vi "OpenCPClior.vi"(11 "CPC port":refnum<visa-resource-name>="COM1") -> (2 "CPC model":string, 3 "dup CPC port":refnum<visa-resource-name>, 10 "read buffer":string)   [LabVIEW 2017]
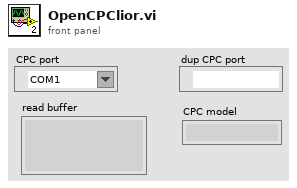
[diagram p1: front panel]
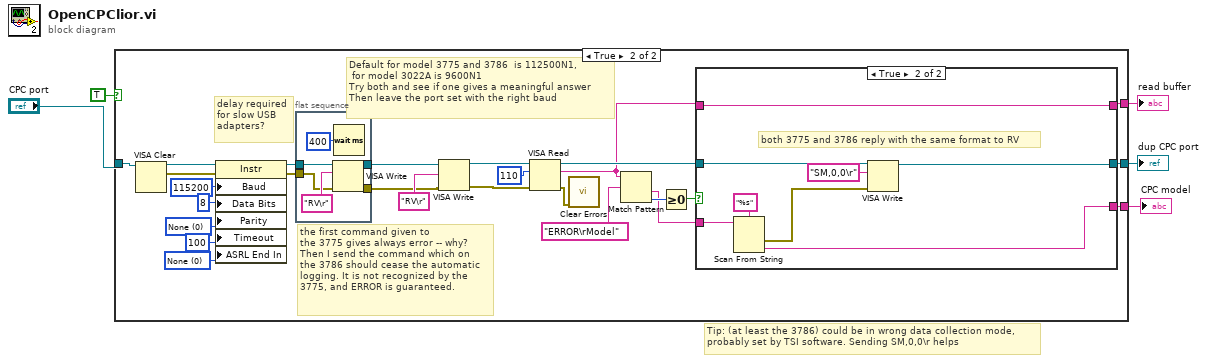
[diagram p0: block diagram]
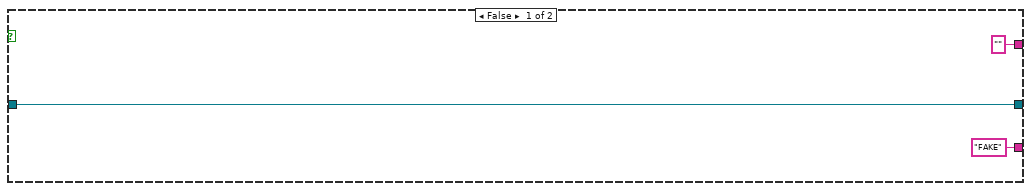
[diagram p2: hidden frame]
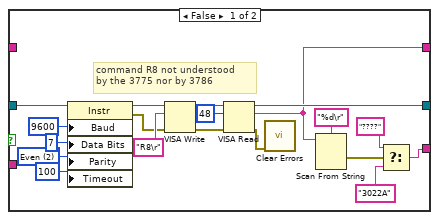
[diagram p3: hidden frame]
diagram:
  # "Tip: (at least the 3786) could be in wrong data collection mode,\nprobably set by TSI software. Sending SM,0,0\\r helps"
  n1 = case shown="True" TRUE {
    tunnel: ["FAKE" ("y") w32] -> w5
    tunnel: ["" ("read buffer") w29] -> w4
    tunnel: "CPC port" -> [w8 w26]
    tunnel: [w8 w25] -> w3
    frame False {
    }
    frame True {
      w9 = u16 0 items=["None", "Last Bit", "TermChar"] ("Serial Settings:End Mode for Reads")
      w19 = u16 0 items=["None", "Odd", "Even", "Mark", "Space"] ("Serial Settings:Parity")
      # "delay required\nfor slow USB\nadapters?"
      # "the first command given to\nthe 3775 gives always error -- why?\nThen I send the command which on\nthe 3786 should cease the automatic\nlogging. It is not recognized by the\n3775, and ERROR is guaranteed."
      # "Default for model 3775 and 3786  is 112500N1,\n for model 3022A is 9600N1\nTry both and see if one gives a meaningful answer\nThen leave the port set with the right baud"
      n2 = VISA Clear(VISA resource name=w26) -> (VISA resource name out=w22:refnum<visa-resource-name>, error out=w17:errorcluster)  [unwired: 1 in]
      n3 = property class="Instr"(reference=w22, error in=w17, "Baud"=u32 115200 ("Serial Settings:Baud Rate"), "Data Bits"=u16 8 ("Serial Settings:Data Bits"), "Parity"=w19, "Timeout"=u32 100 ("General Settings:Timeout Value"), "ASRL End In"=w9) -> (reference out=w23:refnum<visa-resource-name>, error out=w16:errorcluster)
      n4 = flat-sequence {
        tunnel: [w40] -> w24
        tunnel: w23 -> [w38]
        tunnel: w16 -> [w37]
        tunnel: [w36] -> w15
        frame #0 {
          n5 = VISA Write(VISA resource name=w38, write buffer="RV\r", error in (no error)=w37) -> (VISA resource name out=w40:refnum<visa-resource-name>, error out=w36:errorcluster)  [unwired: 1 out]
          n6 = Wait (ms)(milliseconds to wait=u32 400 ("return count")) -> ()  [unwired: 1 out]
        }
      }
      n7 = VISA Write(VISA resource name=w24, write buffer="RV\r", error in (no error)=w15) -> (VISA resource name out=w28:refnum<visa-resource-name>, error out=w14:errorcluster)  [unwired: 1 out]
      n8 = VISA Read(VISA resource name=w28, byte count=u32 110, error in (no error)=w14) -> (VISA resource name out=w33:refnum<visa-resource-name>, read buffer=w30:string, error out=w31:errorcluster)  [unwired: 1 out]
      n9 = call <vilib>:"Clear Errors.vi"("error in (no error)"=w31) -> ()  [unwired: 1 in, 6 out]
      n10 = Match Pattern(string=w30, regular expression="ERROR\rModel" ("y")) -> (after substring=w10:string, offset past match=w11:i32)  [unwired: 3 out]
      n11 = Greater Or Equal To 0?(x=w11) -> (x >= 0?=w12:bool)
      n12 = case shown="True" w12 {
        tunnel: w33 -> [w58 w63]
        tunnel: [w53 w62] -> w25
        tunnel: [w47 w64] -> w32
        tunnel: w30 -> [_ w67]
        tunnel: [w46 w67] -> w29
        tunnel: w10 -> [_ w66]
        frame False {
          w45 = u16 2 items=["None", "Odd", "Even", "Mark", "Space"] ("Serial Settings:Parity")
          # "command R8 not understood \nby the 3775 nor by 3786"
          n13 = property class="Instr"(reference=w58, "Baud"=u32 9600 ("Serial Settings:Baud Rate"), "Data Bits"=u16 7 ("Serial Settings:Data Bits"), "Parity"=w45, "Timeout"=u32 100 ("General Settings:Timeout Value")) -> (reference out=w54:refnum<visa-resource-name>, error out=w41:errorcluster)  [unwired: 1 in]
          n14 = VISA Write(VISA resource name=w54, write buffer="R8\r", error in (no error)=w41) -> (VISA resource name out=w55:refnum<visa-resource-name>, error out=w42:errorcluster)  [unwired: 1 out]
          n15 = VISA Read(VISA resource name=w55, byte count=u32 48, error in (no error)=w42) -> (VISA resource name out=w53:refnum<visa-resource-name>, read buffer=w46:string, error out=w52:errorcluster)  [unwired: 1 out]
          n16 = call <vilib>:"Clear Errors.vi"("error in (no error)"=w52) -> ()  [unwired: 1 in, 6 out]
          n17 = Scan From String(format string="%d\r", input string=w46) -> (error out=w50:errorcluster)  [unwired: 2 in, 4 out]
          n18 = Select(t="????", s=w50, f="3022A" ("y")) -> (s? t:f=w47:string)
        }
        frame True {
          # "both 3775 and 3786 reply with the same format to RV"
          n19 = Scan From String(format string="%s", input string=w66) -> (error out=w61:errorcluster, output 1=w64:string)  [unwired: 2 in, 3 out]
          n20 = VISA Write(VISA resource name=w63, write buffer="SM,0,0\r", error in (no error)=w61) -> (VISA resource name out=w62:refnum<visa-resource-name>)  [unwired: 2 out]
        }
      }
    }
  }
  "dup CPC port" <- w3
  "CPC model" <- w5
  "read buffer" <- w4
